vi "主动发送实时数据直接插入簇 (子VI).vi"() -> (3 "非x？":bool)   [LabVIEW 2016]
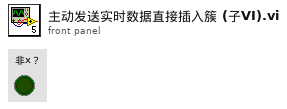
[diagram p1: front panel]
types:
  T1 = cluster{"PH":string[][], "CODCr":string[][], "氨氮":string[][], "CODMn":string[][], "总氮":string[][], "总磷":string[][], "电导率":string[][], "水温":string[][], "DO":string[][], "浊度":string[][], "叶绿素":string[][], "藻密度":string[][]}
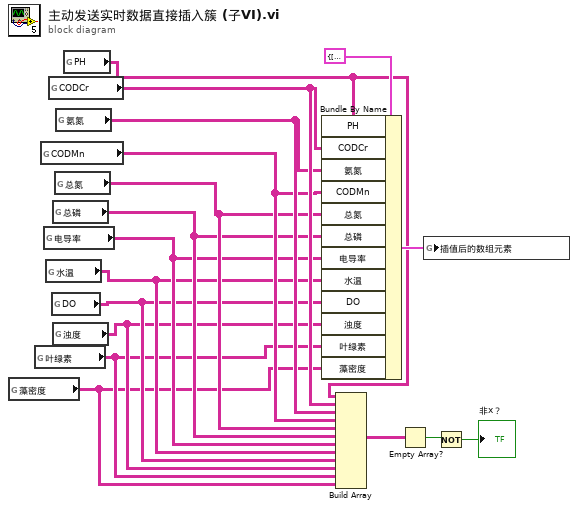
[diagram p0: block diagram]
diagram:
  n1 = global read "全局 所有参数.vi" "藻密度"() -> (w4:string[][])
  n2 = global read "全局 所有参数.vi" "叶绿素"() -> (w5:string[][])
  n3 = global read "全局 所有参数.vi" "CODMn"() -> (w12:string[][])
  n4 = global read "全局 所有参数.vi" "电导率"() -> (w9:string[][])
  n5 = global read "全局 所有参数.vi" "水温"() -> (w8:string[][])
  n6 = global read "全局 所有参数.vi" "CODCr"() -> (w14:string[][])
  n7 = global read "全局 所有参数.vi" "DO"() -> (w7:string[][])
  n8 = global read "全局 所有参数.vi" "总磷"() -> (w10:string[][])
  n9 = global read "全局 所有参数.vi" "浊度"() -> (w6:string[][])
  n10 = global read "全局 所有参数.vi" "总氮"() -> (w11:string[][])
  n11 = global read "全局 所有参数.vi" "氨氮"() -> (w13:string[][])
  n12 = global read "全局 所有参数.vi" "PH"() -> (w15:string[][])
  n13 = Bundle By Name(cluster=T1 {"PH"=[], "CODCr"=[], "氨氮"=[], "CODMn"=[], "总氮"=[], "总磷"=[], "电导率"=[], "水温"=[], "DO"=[], "浊度"=[], "叶绿素"=[], "藻密度"=[]} ("插值后的数组元素"), "PH"=w15, "CODCr"=w14, "氨氮"=w13, "CODMn"=w12, "总氮"=w11, "总磷"=w10, "电导率"=w9, "水温"=w8, "DO"=w7, "浊度"=w6, "叶绿素"=w5, "藻密度"=w4) -> (w17:T1)
  n14 = Build Array(w15, w14, w13, w12, w11, w10, w9, w8, w7, w6, w5, w4) -> (w3:string[][][])
  n15 = Empty Array?(array=w3) -> (empty?=w2:bool)
  n16 = global write "插值后的新数组.vi" "插值后的数组元素"(w17) -> ()
  n17 = Not(x=w2) -> (.not. x?=→"非x？":bool)
